vi "SetTreeSymbols.vi"(6 "Symbol Visibility (unchanged)":enum16{"unchanged", "visible", "invisible"}(ring), 8 "error in (no error)":errorcluster, 9 "Index":i32, 10 "Image":T1, 11 "Tree_LVOOP in":refnum<class "Tree Class.lvclass">) -> (0 "error out":errorcluster, 3 "Tree_LVOOP out":refnum<class "Tree Class.lvclass">)   [LabVIEW 2012, in "Tree Tools.lvlib" / "Tree Class.lvclass"]
uses:
  Tree Class.lvclass
  <vilib>/picture/picture.llb/imagedata.ctl
  Tree Class.lvclass/Tree Class.ctl
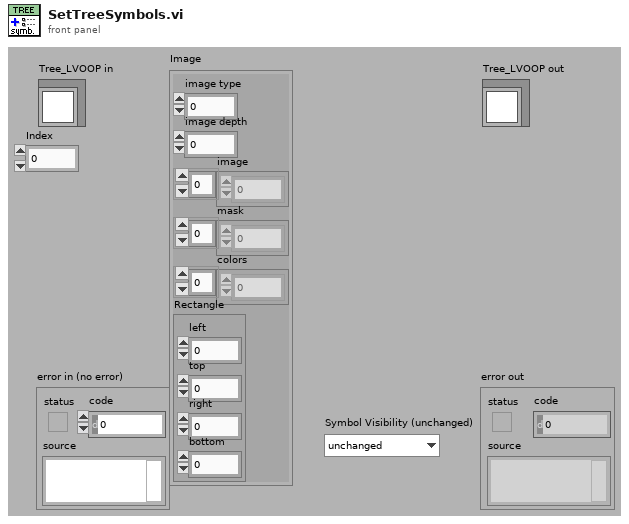
[diagram p1: front panel]
types:
  T1 = typedef "imagedata.ctl" = cluster{"image type":i32, "image depth":i32, "image":u8[], "mask":u8[], "colors":u32[], "Rectangle":cluster{"left":i16, "top":i16, "right":i16, "bottom":i16}}
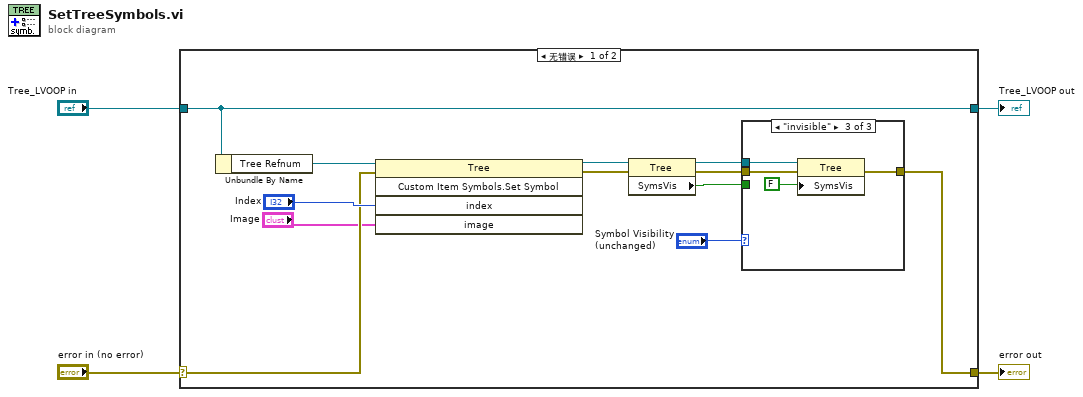
[diagram p0: block diagram]
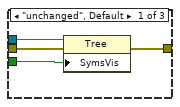
[diagram p2: hidden frame]
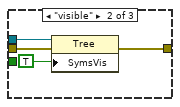
[diagram p3: hidden frame]
diagram:
  n1 = case shown="无错误" "error in (no error)" {
    selector: "error in (no error)" -> [w13 w30]
    tunnel: [w7 w30] -> w3
    tunnel: [w16 w29] -> w1
    tunnel: "Tree_LVOOP in" -> [w16 w29]
    frame No Error {
      n2 = Unbundle By Name(w16) -> ("Tree Refnum"=w15:refnum<vi>)
      n3 = invoke class="Tree" method="Custom Item Symbols.Set Symbol"(reference=w15, error in=w13, "index"="Index", "image"="Image") -> (reference out=w11:refnum<vi>, error out=w5:errorcluster)  [unwired: 1 in, 3 out]
      n4 = property class="Tree"(reference=w11, error in=w5) -> (reference out=w10:refnum<vi>, error out=w6:errorcluster, "SymsVis"=w8:bool)
      n5 = case shown="\"invisible\"" "Symbol Visibility (unchanged)" {
        tunnel: w10 -> [w20 w24 w28]
        tunnel: w8 -> [w19 _ _]
        tunnel: [w18 w22 w26] -> w7
        tunnel: w6 -> [w17 w21 w25]
        frame "unchanged", Default {
          n6 = property class="Tree"(reference=w20, error in=w17, "SymsVis"=w19) -> (error out=w18:errorcluster)  [unwired: 1 out]
        }
        frame "visible" {
          n7 = property class="Tree"(reference=w24, error in=w21, "SymsVis"=TRUE ("Visible Items:Symbols Visible")) -> (error out=w22:errorcluster)  [unwired: 1 out]
        }
        frame "invisible" {
          n8 = property class="Tree"(reference=w28, error in=w25, "SymsVis"=FALSE ("Visible Items:Symbols Visible")) -> (error out=w26:errorcluster)  [unwired: 1 out]
        }
      }
    }
    frame Error {
    }
  }
  "error out" <- w3
  "Tree_LVOOP out" <- w1
